vi "writeToXML.vi"(8 "error in (no error)":errorcluster, 10 "Class Label":string="AzElError", 11 "AzElError in":refnum<class "AzElError.lvclass">) -> (0 "error out":errorcluster, 2 "XML out":string="<>\n  <azError>0</azError>\n  <elError>0</elError>\n</>", 3 "AzElError out":refnum<class "AzElError.lvclass">)   [LabVIEW 2014, in "TCSDataDefinitions.lvlib" / "TCSPublicStatus.lvlib" / "PointingPositions.lvlib" / "AzElError.lvclass"]
uses:
  AzElError.lvclass
  <userlib>/Common/UnitsAndXML/FlattenItemWithUnitToXML/FlattenPlaneAngleToXML/PlaneAngleUnit.ctl
  AzElError.lvclass/AzElError.ctl
  <userlib>/Common/UnitsAndXML/UnitsAndXML.lvlib
  <userlib>/Common/XML/XMLGenerator/XMLGenerator.lvclass
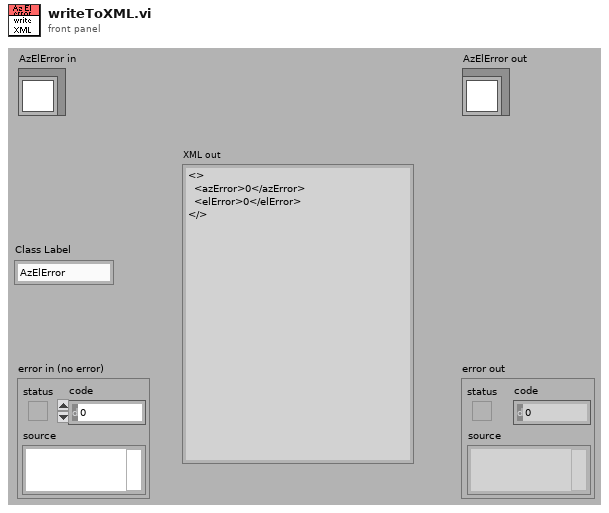
[diagram p1: front panel]
types:
  T1 = typedef "UnitsAndXML.lvlib/PlaneAngleUnit.ctl" = enum16{"rad", "deg", "'", "\""}
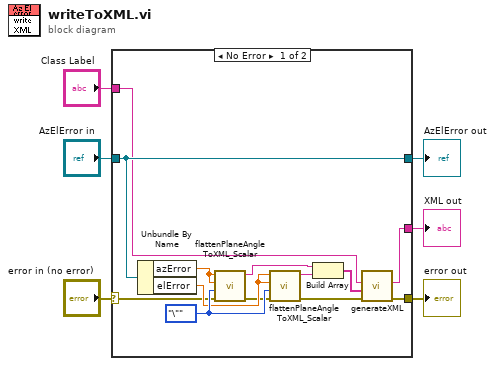
[diagram p0: block diagram]
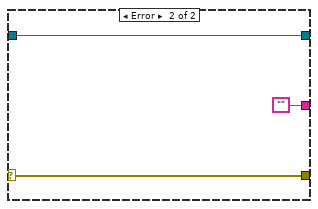
[diagram p2: hidden frame]
diagram:
  n1 = case shown="No Error" "error in (no error)" {
    selector: "error in (no error)" -> [w14 w22]
    tunnel: [w12 w22] -> w5
    tunnel: [w19 w21] -> w3
    tunnel: "AzElError in" -> [w19 w21]
    tunnel: [w11 ""] -> w2
    tunnel: "Class Label" -> [w8 _]
    frame No Error {
      w17 = PlaneAngleUnit."\"" ("planeAngleUnitInXML")
      n2 = Unbundle By Name(w19) -> ("azError"=w18:dbl[unit], "elError"=w16:dbl[unit])
      n3 = call <userlib>:"flattenPlaneAngleToXML_Scalar.vi"("error in (no error)"=w14, "planeAngleUnitInXML"=w17, "planeAngleAgain"=w18, "planeAngle"=w18) -> ("error out"=w15:errorcluster, "xmlString"=w10:string)  [unwired: 6 in]
      n4 = call <userlib>:"flattenPlaneAngleToXML_Scalar.vi"("error in (no error)"=w15, "planeAngleUnitInXML"=w17, "planeAngleAgain"=w16, "planeAngle"=w16) -> ("error out"=w13:errorcluster, "xmlString"=w9:string)  [unwired: 6 in]
      n5 = Build Array(w10, w9) -> (w7:string[])
      n6 = call <userlib>:"generateXML.vi"("error in"=w13, "childrenXML"=w7, "elementName"=w8) -> ("error out"=w12:errorcluster, "XML out"=w11:string)  [unwired: 6 in, 1 out]
    }
    frame Error {
    }
  }
  "error out" <- w5
  "AzElError out" <- w3
  "XML out" <- w2
